vi "Main.vi"(11 "Module Admin":refnum<class "Delacor_lib_QMH_Cloneable Module Admin.lvclass">) -> ()   [LabVIEW 2020, in "Osciloscope.lvlib"]
doc: "This template is based off of the Queued Message Handler design pattern and the Queued Message Handler project template that ships with LabVIEW.\n\nThe main difference is that the queue is private to this module and communication between modules is performed via Broadcast and Request events.\n\nRequest events are wrapped in public API methods and are handled in the Event Handling Loop (EHL) of this VI. Any module can register for Broadcast events sent by this module. The EHL generates messages based on user interface actions.\n\nThe Message Handling Loop (MHL) processes messages generated by the EHL, or by other messages. The messages are string values, so new messages can be added easily to the Message Cases case structure in the MHL. Each message cluster can also provide an optional value for Message Data, which is a variant that can be converted to whatever message-specific data is required.\n_____\nBased on DQMH Project Template 6.0.0.91."
uses:
  Osciloscope.lvlib
  <vilib>/Delacor/Delacor QMH/Libraries/Cloneable Module Admin_class/Delacor_lib_QMH_Cloneable Module Admin.lvclass
  C:/Program Files (x86)/National Instruments/LabVIEW 2020/vi.lib/Delacor/Delacor QMH/Libraries/Module Admin_class/Delacor_lib_QMH_Module Admin.lvclass
  Module Data--cluster.ctl
  Class/Implementaciones/OsciloscopeClass/OsciloscopeClass.lvclass
  <vilib>/Delacor/Delacor QMH/Libraries/Message Queue_class/Delacor_lib_QMH_Message Queue.lvclass/Delacor_lib_QMH_Message Queue.ctl
  <vilib>/Delacor/Delacor QMH/Libraries/Cloneable Module Admin_class/Delacor_lib_QMH_Cloneable Module Admin.lvclass/Delacor_lib_QMH_Cloneable Module Admin.ctl
  Stop Argument--cluster.ctl
  <vilib>/Delacor/Delacor QMH/Libraries/Module Admin_class/Delacor_lib_QMH_Module Admin.lvclass/Delacor_lib_QMH_Module Admin.ctl
  Set Com Port Argument--cluster.ctl
  Inizializate Argument--cluster.ctl
  Init Osciloscope Argument--cluster.ctl
  TypeDefs/InitializeOsciloscope--cluster.ctl
  Close Osciloscope Argument--cluster.ctl
  Auto Setup Osciloscope Argument--cluster.ctl
  Configure Channel Argument--cluster.ctl
  TypeDefs/ConfigurateCahnnel--cluster.ctl
  Reset Osciloscope Argument--cluster.ctl
  Read Waveform Osciloscope Argument--cluster.ctl
  TypeDefs/ReadWaveform--cluster.ctl
  Read Waveform Osciloscope (Reply Payload)--cluster.ctl
  Read Measurement Osciloscope Argument--cluster.ctl
  TypeDefs/ReadMeasurementIn--cluster.ctl
  Read Measurement Osciloscope (Reply Payload)--cluster.ctl
  TypeDefs/ReadMeasurementOut--cluster.ctl
  Read 2 Measurement Channels Osciloscope Argument--cluster.ctl
  TypeDefs/Read2channelsIn--cluster.ctl
  Read 2 Measurement Channels Osciloscope (Reply Payload)--cluster.ctl
  TypeDefs/Read2ChannlesOut.ctl
  <vilib>/Utility/miscctls.llb/LVPointTypeDef.ctl
  Class/Implementaciones/OsciloscopeClass/OsciloscopeClass.lvclass/OsciloscopeClass.ctl
  <vilib>/Delacor/Delacor QMH/Libraries/Message Queue_class/Delacor_lib_QMH_Enqueue Message (Single).vi
  <vilib>/Delacor/Delacor QMH/Libraries/Cloneable Module Admin_class/Delacor_lib_QMH_Get Module ID.vi
  <vilib>/Delacor/Delacor QMH/Libraries/Module Admin_class/Delacor_lib_QMH_Get External Launch.vi
  Class/Implementaciones/OsciloscopeClass/Write Com Port.vi
  <vilib>/Utility/error.llb/Error Cluster From Error Code.vi
  <vilib>/ErrorRing/Error Ring.xnode
  <vilib>/Delacor/Delacor QMH/Libraries/Message Queue_class/Delacor_lib_QMH_Message Queue.lvclass
panel:
  out "error out":errorcluster
  out "Status":string
  in  "Simulate EHL Error":bool
  in  "Simulate MHL Error":bool
  # "Other QMH Modules communicate with this Module via its Public API (wrappers for its Request Events).\n\nThis Module communicates with other Modules via its Broadcast Events.\nAny module that wants to get these messages, just registers for this module's Broadcast events."
  # "This template is for the Delacor Modified Queued Message Handler design pattern.\n\nSee the block diagram for more information on how to use this template."
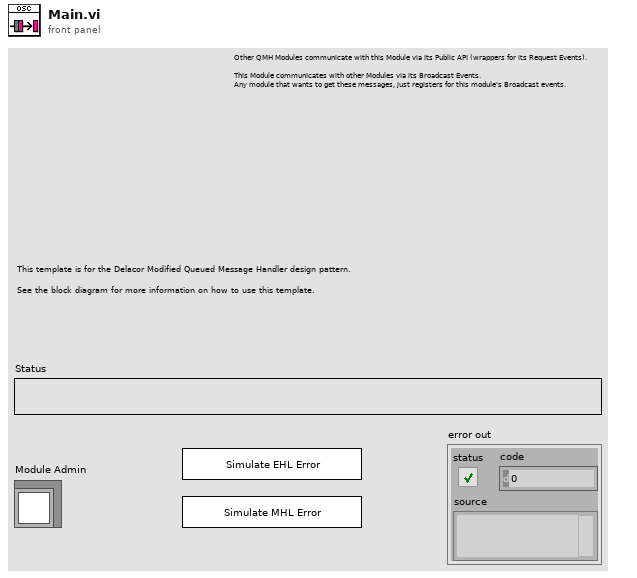
[diagram p1: front panel]
types:
  T1 = typedef "Osciloscope.lvlib/Request Events--cluster.ctl" = cluster{"Stop Module":refnum<user-event>, "Show Panel":refnum<user-event>, "Hide Panel":refnum<user-event>, "Show Diagram":refnum<user-event>, "Get Module Execution Status":refnum<user-event>, "Set Com Port":refnum<user-event>, "Inizializate":refnum<user-event>, "Init Osciloscope":refnum<user-event>, "Close Osciloscope":refnum<user-event>, "Auto Setup Osciloscope":refnum<user-event>, "Configure Channel":refnum<user-event>, "Reset Osciloscope":refnum<user-event>, "Read Waveform Osciloscope":refnum<user-event>, "Read Measurement Osciloscope":refnum<user-event>, "Read 2 Measurement Channels Osciloscope":refnum<user-event>}
  T2 = typedef "Osciloscope.lvlib/Module Data--cluster.ctl" = cluster{"Status":string, "OsciloscopeClass.lvclass":refnum<class "OsciloscopeClass.lvclass">}
  T3 = enum32{"invalid lock state", "Not Locked", "Locked (No Password)", "Password-protected"}
  T4 = typedef "Osciloscope.lvlib/Stop Argument--cluster.ctl" = cluster{"Module ID":i32, "Origin":string, "Exit via Stop Module Req?":bool, "Wait for Module to stop?":bool}
  T5 = typedef "Osciloscope.lvlib/Set Com Port Argument--cluster.ctl" = cluster{"Module ID":i32, "Com Port":refnum<visa-resource-name>}
  T6 = typedef "Osciloscope.lvlib/Inizializate Argument--cluster.ctl" = cluster{"Module ID":i32, "Osciloscope":string}
  T7 = typedef "Osciloscope.lvlib/Init Osciloscope Argument--cluster.ctl" = cluster{"Module ID":i32, "Boolean":bool, "Initialize--cluster":T8}
  T8 = typedef "InitializeOsciloscope--cluster.ctl" = cluster{"TEKTRONIX-INITIALIZE":cluster{"ID Query? (T: Yes)":bool, "Reset? (T: Yes)":bool, "Serial-Configuration":cluster{"Baud Rate":u32, "Parity":u16, "Stop Bits":u16, "Flow Control":u16}}, "EDU-X-1200A- INITIALIZE":cluster{"Reset (True)":bool, "ID Query (True)":bool}}
  T9 = typedef "Osciloscope.lvlib/Close Osciloscope Argument--cluster.ctl" = cluster{"Module ID":i32, "Boolean":bool}
  T10 = typedef "Osciloscope.lvlib/Auto Setup Osciloscope Argument--cluster.ctl" = cluster{"Module ID":i32, "Boolean":bool}
  T11 = typedef "Osciloscope.lvlib/Configure Channel Argument--cluster.ctl" = cluster{"Module ID":i32, "Configurate Channel--cluster":T12}
  T12 = typedef "ConfigurateCahnnel--cluster.ctl" = cluster{"Tektronix":cluster{"Enable Channel (True)":bool, "Channel (0: Channel 1)":i32, "Vertical Coupling (1: DC)":i32, "Probe Attenuation (10: 10X)":i32, "Vertical Range (10.0 V/div)":dbl, "Vertical Offset (0.0 divs)":dbl, "Bandwidth (0: MAX Bandwidth)":i32}, "EDU-X-1002A":cluster{"Vertical Scale (5.0 V)":dbl, "Impedance (0: 1 MOhm)":i32, "Channel Name (0: Channel 1)":i32, "Coupling (1: DC)":i32, "Vertical Range (40.0 V)":dbl, "Vertical Offset (0.0)":dbl, "Probe Attenuation (1.0)":dbl, "Vertical Setting (1: Vertical Range)":i32}}
  T13 = typedef "Osciloscope.lvlib/Reset Osciloscope Argument--cluster.ctl" = cluster{"Module ID":i32, "Boolean":bool}
  T14 = typedef "Osciloscope.lvlib/Read Waveform Osciloscope Argument--cluster.ctl" = cluster{"Module ID":i32, "ReadWaveform":T15, "Wait Notifier":refnum<notifier>, "wait for reply":bool}
  T15 = typedef "ReadWaveform--cluster.ctl" = cluster{"TEKTRONIX READ-WAVEFORM 2":cluster{"Source (0: Channel 1)":u16, "Timeout (10000 ms) 2":u32}, "EDU-X-1200A- READ-WAVEFORM":cluster{"Bind Source Channel (2: None)":i32, "Timeout (10000 ms)":u32, "Source Channel (0: Channel 1)":i32}}
  T16 = typedef "Osciloscope.lvlib/Read Measurement Osciloscope Argument--cluster.ctl" = cluster{"Module ID":i32, "Read Measurement In":T17, "Wait Notifier":refnum<notifier>, "wait for reply":bool}
  T17 = typedef "ReadMeasurementIn--cluster.ctl" = cluster{"TEKTRONIX- READ-IN":cluster{"Channel (1: Channel 1)":i32, "Measurement Type (0: Frequency)":i32}, "EDU-X-1200A- READ-IN":cluster{"Slope Type (0: Positive)":i32, "Measurement Type (0: Peak-Peak)":i32, "Occurrence Value (1)":i32, "Vertical Cross Value (0)":dbl}}
  T18 = typedef "Osciloscope.lvlib/Read 2 Measurement Channels Osciloscope Argument--cluster.ctl" = cluster{"Module ID":i32, "Read 2 channels In":T19, "Wait Notifier":refnum<notifier>, "wait for reply":bool}
  T19 = typedef "Read2channelsIn--cluster.ctl" = cluster{"TEKTRONIX- READ-CHANNELS-IN":cluster{"Channel 1 (1: Channel 1)":i32, "Channel 2 (2: Channel 2)":i32, "Measurement Type (0: Phase)":i32}, "EDU-X-1200A- READ-CHANNELS-IN":cluster{"Timeout (10000 ms)":u32, "Channels":i32[]}}
  T20 = typedef "LVPointTypeDef.ctl" = cluster{"Horizontal":i16, "Vertical":i16}
  T21 = enum32{"Invalid", "Standard", "Closed", "Hidden", "Minimized", "Maximized"}
  T22 = typedef "Osciloscope.lvlib/Read Waveform Osciloscope (Reply Payload)--cluster.ctl" = cluster{"Waveform Graph":dbl[], "Read Waveform Osciloscope_error":errorcluster}
  T23 = typedef "Osciloscope.lvlib/Read Measurement Osciloscope (Reply Payload)--cluster.ctl" = cluster{"Read measurement Out":T24, "Read Measurement Osciloscope_error":errorcluster}
  T24 = typedef "ReadMeasurementOut--cluster.ctl" = cluster{"Tektronix-1200A-READ-OUT":cluster{"Units":string, "Measurement":dbl}, "EDU-X-1200A- READ-OUT":cluster{"Measurement":dbl}}
  T25 = typedef "Osciloscope.lvlib/Read 2 Measurement Channels Osciloscope (Reply Payload)--cluster.ctl" = cluster{"Read 2 channels Out":T26, "Read 2 Measurement Channels Osciloscope_error":errorcluster}
  T26 = typedef "Read2ChannlesOut.ctl" = cluster{"TEKTRONIX READ-CHANNELS-OUT ":cluster{"Units":string, "Measurement":dbl}, "EDU-X-1200A- READ-CHANNELS-OUT":cluster{"Measurements":dbl[]}}
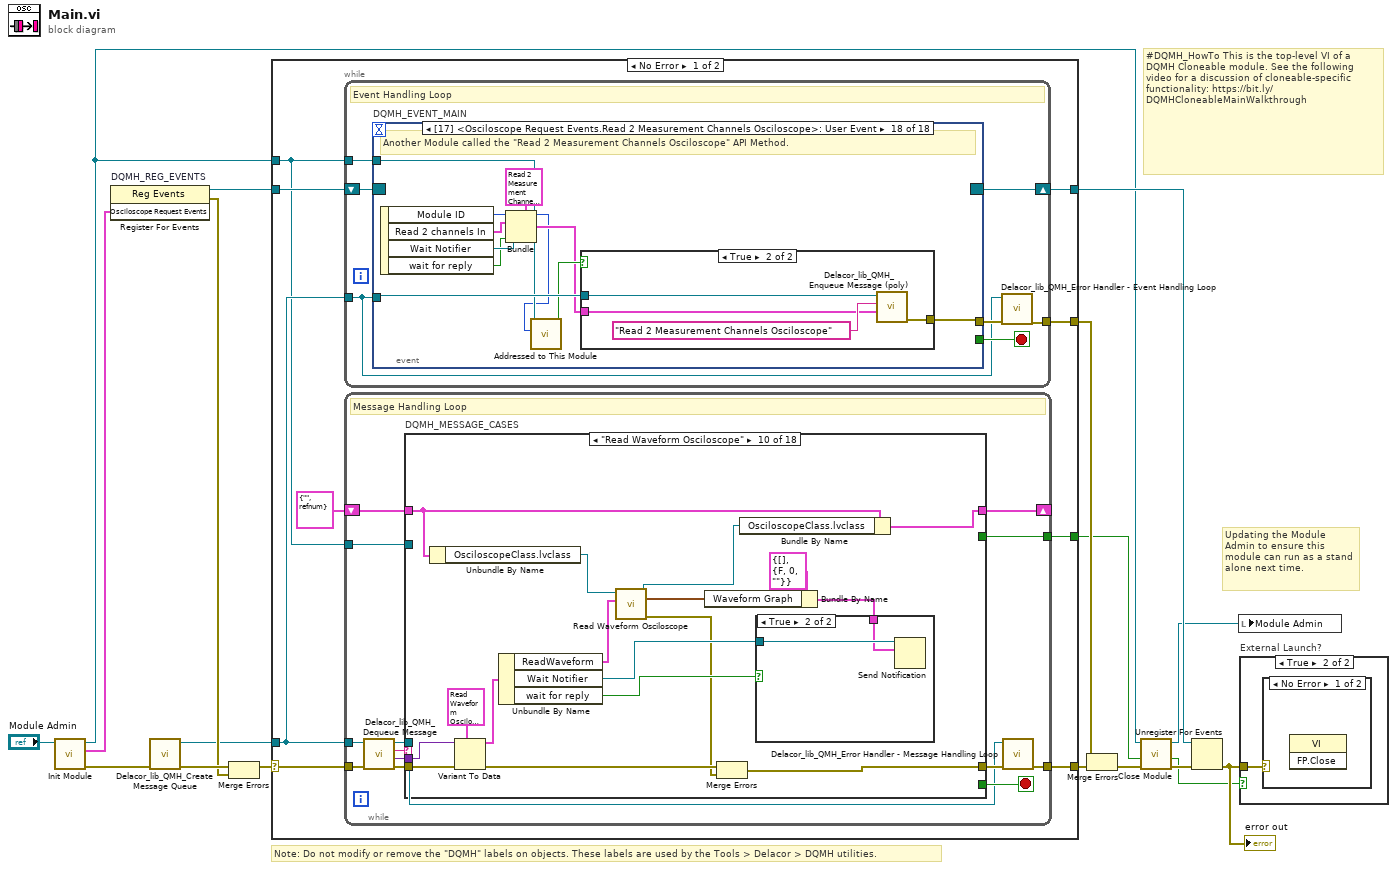
[diagram p0: block diagram]
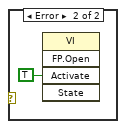
[diagram p3: hidden frame]
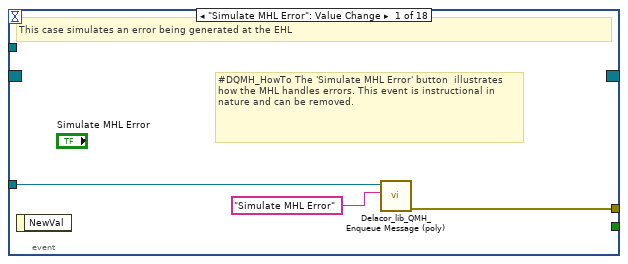
[diagram p4: hidden frame]
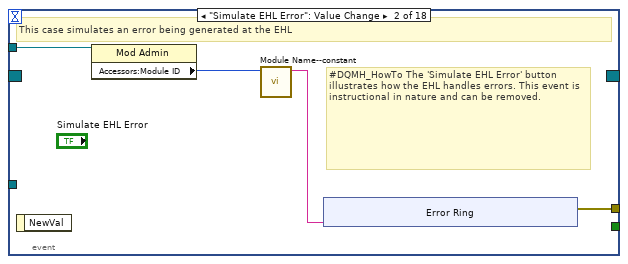
[diagram p5: hidden frame]
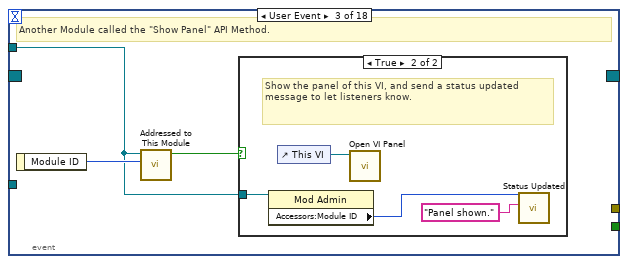
[diagram p6: hidden frame]
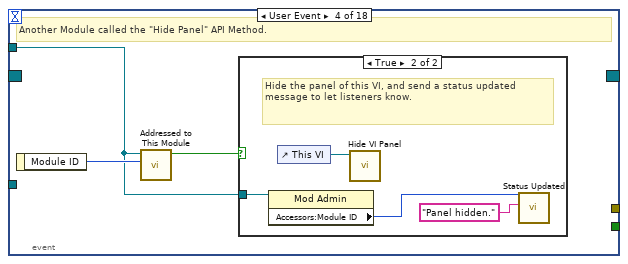
[diagram p8: hidden frame]
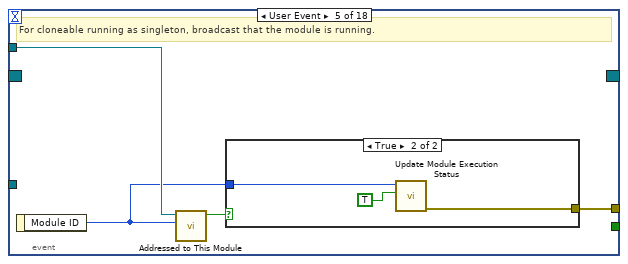
[diagram p10: hidden frame]
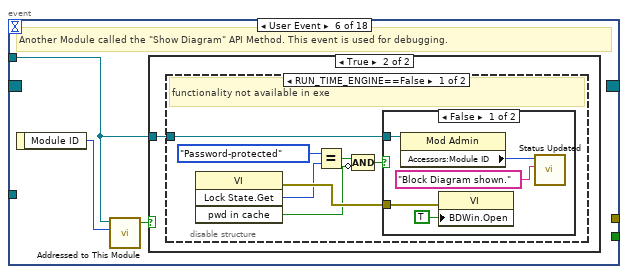
[diagram p12: hidden frame]
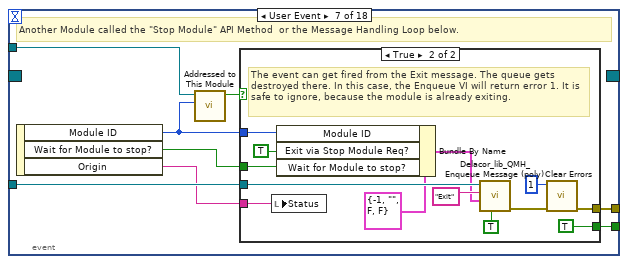
[diagram p16: hidden frame]
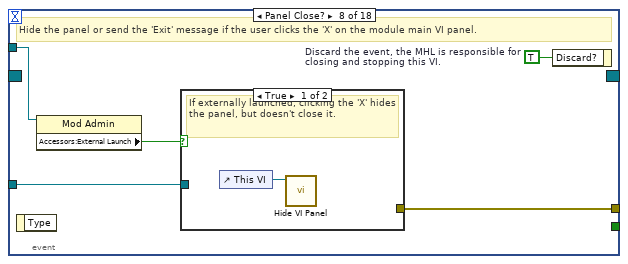
[diagram p18: hidden frame]
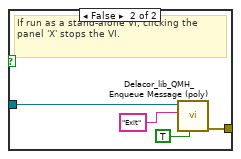
[diagram p19: hidden frame]
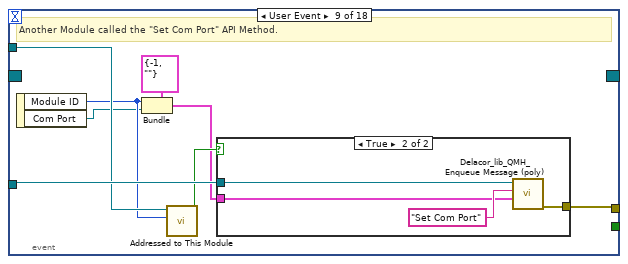
[diagram p20: hidden frame]
diagram:
  # "#DQMH_HowTo This is the top-level VI of a DQMH Cloneable module. See the following video for a discussion of cloneable-specific functionality: https://bit.ly/DQMHCloneableMainWalkthrough"
  # "Note: Do not modify or remove the \"DQMH\" labels on objects. These labels are used by the Tools > Delacor > DQMH utilities."
  # "Updating the Module Admin to ensure this module can run as a stand alone next time."
  n1 = call "Init Module.vi"("Cloneable Module Admin in"="Module Admin") -> ("error out"=w15:errorcluster, "Osciloscope Request Events"=w7:T1, "Cloneable Module Admin out"=w4:refnum<class "Delacor_lib_QMH_Cloneable Module Admin.lvclass">)  [unwired: 8 in]
  n2 = register-events "DQMH_REG_EVENTS"(w7) -> (reference out=w8:refnum<event-registration>, error out=w10:errorcluster)  [unwired: 2 in]
  n3 = call <vilib>:"Delacor_lib_QMH_Create Message Queue.vi"("error in"=w15) -> ("error out"=w12:errorcluster, "Message Queue"=w6:refnum<class "Delacor_lib_QMH_Message Queue.lvclass">)  [unwired: 9 in]
  n4 = Merge Errors(w12, w10) -> (w11:errorcluster)
  n5 = case shown="No Error" w11 {
    selector: w11 -> [w25 w475]
    tunnel: [w27 w474] -> w16
    tunnel: [w24 w482] -> w9
    tunnel: w8 -> [w22 w482]
    tunnel: w6 -> [w21 w473]
    tunnel: [w26 _] -> w17
    tunnel: w4 -> [w20 w478]
    tunnel: [w19 _] -> w2
    frame No Error {
      n6 = while {
        tunnel: w21 -> [w28]
        shift-right: [w31] -> w24
        shift-left: w22 -> [w32]
        tunnel: [w33] -> w26
        tunnel: w20 -> [w29]
        stop <- w30 stop-if-true
        # "Event Handling Loop"
        n7 = event "DQMH_EVENT_MAIN" shown="[17] <Osciloscope Request Events.Read 2 Measurement Channels Osciloscope>: User Event" {
          selector: w32 -> [_ _ _ _ _ _ _ _ _ _ _ _ _ _ _ _ _ _]
          dyn-events: [_ _ _ _ _ _ _ _ _ _ _ _ _ _ _ _ _ _] -> w31
          timeout: _ -> [_ _ _ _ _ _ _ _ _ _ _ _ _ _ _ _ _ _]
          tunnel: [_ _ _ _ _ _ w89 _ _ _ _ _ _ _ _ _ _ _] -> w30
          tunnel: w28 -> [w36 _ _ _ _ _ w92 w108 w124 w136 w149 w161 w173 w185 w197 w211 w225 w239]
          tunnel: [w37 w41 _ _ w66 _ w93 w111 w117 w129 w142 w154 w166 w178 w190 w202 w216 w230] -> w34
          tunnel: w29 -> [_ w40 w49 w56 w64 w70 w91 w109 w122 w134 w147 w159 w171 w183 w195 w209 w223 w237]
          event "Simulate MHL Error": Value Change {
            # "#DQMH_HowTo The 'Simulate MHL Error' button  illustrates how the MHL handles errors. This event is instructional in nature and can be removed."
            # "This case simulates an error being generated at the EHL"
            n8 = event-data() -> ()  [unwired: 1 in, 1 out]
            n9 = call-poly <vilib>:"Delacor_lib_QMH_Enqueue Message (poly).vi"("Message"="Simulate MHL Error", "Message Queue in"=w36) -> ("error out"=w37:errorcluster)  [unwired: 8 in, 1 out]
          }
          event "Simulate EHL Error": Value Change {
            # "#DQMH_HowTo The 'Simulate EHL Error' button  illustrates how the EHL handles errors. This event is instructional in nature and can be removed."
            # "This case simulates an error being generated at the EHL"
            n10 = event-data() -> ()  [unwired: 1 in, 1 out]
            n11 = property class="Mod Admin"(reference=w40) -> ("Accessors:Module ID"=w39:i32)  [unwired: 1 in, 2 out]
            n12 = call "Module Name--constant.vi"("Module ID"=w39) -> ("Module Name"=w38:string)  [unwired: 10 in]
            n13 = xnode "Error Ring"("parameter 0"=w38) -> ("error out"=w41:errorcluster)
          }
          event User Event {
            # "Another Module called the \"Show Panel\" API Method."
            n14 = event-data() -> ("Module ID"=w50:i32)  [unwired: 1 in]
            n15 = call "Addressed to This Module.vi"("Module ID from Argument"=w50, "Module Admin"=w49) -> ("Addressed to this instance?"=w51:bool)  [unwired: 8 in, 1 out]
            n16 = case shown="True" w51 {
              tunnel: w49 -> [_ w53]
              frame False {
              }
              frame True {
                # "Show the panel of this VI, and send a status updated message to let listeners know."
                n17 = property class="Mod Admin"(reference=w53) -> ("Accessors:Module ID"=w52:i32)  [unwired: 1 in, 2 out]
                n18 = control-ref of="This VI"() -> (w55:refnum<vi>)
                n19 = call "Open VI Panel.vi"("VI"=w55) -> ()  [unwired: 10 in, 1 out]
                n20 = call "Status Updated.vi"("Status"="Panel shown." ("format string"), "Module ID"=w52) -> ()  [unwired: 9 in, 1 out]
              }
            }
          }
          event User Event {
            # "Another Module called the \"Hide Panel\" API Method."
            n21 = event-data() -> ("Module ID"=w57:i32)  [unwired: 1 in]
            n22 = call "Addressed to This Module.vi"("Module ID from Argument"=w57, "Module Admin"=w56) -> ("Addressed to this instance?"=w58:bool)  [unwired: 8 in, 1 out]
            n23 = case shown="True" w58 {
              tunnel: w56 -> [_ w60]
              frame False {
              }
              frame True {
                # "Hide the panel of this VI, and send a status updated message to let listeners know."
                n24 = property class="Mod Admin"(reference=w60) -> ("Accessors:Module ID"=w59:i32)  [unwired: 1 in, 2 out]
                n25 = control-ref of="This VI"() -> (w62:refnum<vi>)
                n26 = call "Hide VI Panel.vi"("VI"=w62) -> ()  [unwired: 10 in, 1 out]
                n27 = call "Status Updated.vi"("Status"="Panel hidden." ("format string"), "Module ID"=w59) -> ()  [unwired: 9 in, 1 out]
              }
            }
          }
          event User Event {
            # "For cloneable running as singleton, broadcast that the module is running."
            n28 = event-data() -> ("Module ID"=w63:i32)  [unwired: 1 in]
            n29 = call "Addressed to This Module.vi"("Module ID from Argument"=w63, "Module Admin"=w64) -> ("Addressed to this instance?"=w65:bool)  [unwired: 8 in, 1 out]
            n30 = case shown="True" w65 {
              tunnel: [_ w69] -> w66
              tunnel: w63 -> [_ w68]
              frame False {
              }
              frame True {
                n31 = call "Update Module Execution Status.vi"("Running?"=TRUE, "Module ID"=w68) -> ("error out"=w69:errorcluster)  [unwired: 9 in]
              }
            }
          }
          event User Event {
            # "Another Module called the \"Show Diagram\" API Method. This event is used for debugging."
            n32 = event-data() -> ("Module ID"=w71:i32)  [unwired: 1 in]
            n33 = call "Addressed to This Module.vi"("Module ID from Argument"=w71, "Module Admin"=w70) -> ("Addressed to this instance?"=w72:bool)  [unwired: 8 in, 1 out]
            n34 = case shown="True" w72 {
              tunnel: w70 -> [_ w73]
              frame False {
              }
              frame True {
                n35 = disable-structure shown="RUN_TIME_ENGINE==False" {
                  disable-tunnel: w73 -> [w74 _]
                  frame condition #0 (active) {
                    # "functionality not available in exe"
                    n36 = invoke class="VI" method="Lock State.Get"() -> (error out=w80:errorcluster, "Get Lock State"=w79:T3, "pwd in cache"=w76:bool)  [unwired: 4 in, 1 out]
                    n37 = Equal?(x=T3."Password-protected", y=w79) -> (x = y?=w77:bool)
                    n38 = Compound Arithmetic op=AND(w77, invert w76) -> (w75:bool)
                    n39 = case shown="False" w75 {
                      tunnel: w80 -> [w85 _]
                      tunnel: w74 -> [w82 _]
                      frame False {
                        n40 = property class="Mod Admin"(reference=w82) -> ("Accessors:Module ID"=w81:i32)  [unwired: 1 in, 2 out]
                        n41 = property class="VI"(error in=w85, "BDWin.Open"=TRUE ("Block Diagram Window:Open")) -> ()  [unwired: 1 in, 2 out]
                        n42 = call "Status Updated.vi"("Status"="Block Diagram shown." ("format string"), "Module ID"=w81) -> ()  [unwired: 9 in, 1 out]
                      }
                      frame True {
                        # "Password-protected VI, and the password is not in the cache. Do not show the diagram."
                      }
                    }
                  }
                  frame condition #1 {
                  }
                }
              }
            }
          }
          event User Event {
            # "Another Module called the \"Stop Module\" API Method  or the Message Handling Loop below."
            n43 = event-data() -> ("Module ID"=w87:i32, "Wait for Module to stop?"=w88:bool, "Origin"=w86:string)  [unwired: 1 in]
            n44 = call "Addressed to This Module.vi"("Module ID from Argument"=w87, "Module Admin"=w91) -> ("Addressed to this instance?"=w90:bool)  [unwired: 8 in, 1 out]
            n45 = case shown="True" w90 {
              tunnel: [_ w105] -> w93
              tunnel: w92 -> [_ w101]
              tunnel: [_ TRUE] -> w89
              tunnel: w88 -> [_ w96]
              tunnel: w87 -> [_ w98]
              tunnel: w86 -> [_ w94]
              frame False {
              }
              frame True {
                # "The event can get fired from the Exit message. The queue gets destroyed there. In this case, the Enqueue VI will return error 1. It is safe to ignore, because the module is already exiting."
                n46 = local write "Status"(w94) -> ()
                n47 = Bundle By Name(cluster=T4 {"Module ID"=-1, "Origin"="", "Exit via Stop Module Req?"=FALSE, "Wait for Module to stop?"=FALSE} ("Stop Argument"), "Module ID"=w98, "Exit via Stop Module Req?"=TRUE, "Wait for Module to stop?"=w96) -> (w95:T4)
                n48 = call-poly <vilib>:"Delacor_lib_QMH_Enqueue Message (poly).vi"("Priority Message? (F)"=TRUE, "Message Data"=w95, "Message"="Exit", "Message Queue in"=w101) -> ("error out"=w106:errorcluster)  [unwired: 6 in, 1 out]
                n49 = call <vilib>:"Clear Errors.vi"("error in (no error)"=w106, "specific error code to clear (0: all)"=1) -> ("error out"=w105:errorcluster)  [unwired: 4 in, 1 out]
              }
            }
          }
          event Panel Close? {
            w110 = TRUE  # Discard the event, the MHL is responsible for closing and stopping this VI.
            # "Hide the panel or send the 'Exit' message if the user clicks the 'X' on the module main VI panel."
            n50 = event-data() -> ()  [unwired: 1 in, 1 out]
            n51 = property class="Mod Admin"(reference=w109) -> ("Accessors:External Launch"=w107:bool)  [unwired: 1 in, 2 out]
            n52 = case shown="True" w107 {
              tunnel: w108 -> [_ w115]
              tunnel: [_ w116] -> w111
              frame True {
                # "If externally launched, clicking the 'X' hides the panel, but doesn't close it."
                n53 = control-ref of="This VI"() -> (w112:refnum<vi>)
                n54 = call "Hide VI Panel.vi"("VI"=w112) -> ()  [unwired: 10 in, 1 out]
              }
              frame False {
                # "If run as a stand-alone VI, clicking the panel 'X' stops the VI."
                n55 = call-poly <vilib>:"Delacor_lib_QMH_Enqueue Message (poly).vi"("Priority Message? (F)"=TRUE, "Message"="Exit", "Message Queue in"=w115) -> ("error out"=w116:errorcluster)  [unwired: 7 in, 1 out]
              }
            }
            n56 = event-data("Discard?"=w110) -> ()  [unwired: 1 in, 1 out]
          }
          event User Event {
            # "Another Module called the \"Set Com Port\" API Method."
            n57 = event-data() -> ("Module ID"=w119:i32, "Com Port"=w118:refnum<visa-resource-name>)  [unwired: 1 in]
            n58 = Bundle(cluster=T5 {"Module ID"=-1, "Com Port"=""} ("Set Com Port Argument"), "Module ID"=w119, "Com Port"=w118) -> (w120:T5)
            n59 = call "Addressed to This Module.vi"("Module ID from Argument"=w119, "Module Admin"=w122) -> ("Addressed to this instance?"=w123:bool)  [unwired: 8 in, 1 out]
            n60 = case shown="True" w123 {
              tunnel: w124 -> [_ w128]
              tunnel: w120 -> [_ w126]
              tunnel: [_ w125] -> w117
              frame False {
              }
              frame True {
                n61 = call-poly <vilib>:"Delacor_lib_QMH_Enqueue Message (poly).vi"("Message Data"=w126, "Message"="Set Com Port", "Message Queue in"=w128) -> ("error out"=w125:errorcluster)  [unwired: 7 in, 1 out]
              }
            }
          }
          event User Event {
            # "Another Module called the \"Inizializate\" API Method."
            n62 = event-data() -> ("Module ID"=w131:i32, "Osciloscope"=w130:string)  [unwired: 1 in]
            n63 = Bundle(cluster=T6 {"Module ID"=-1, "Osciloscope"=""} ("Inizializate Argument"), "Module ID"=w131, "Osciloscope"=w130) -> (w132:T6)
            n64 = call "Addressed to This Module.vi"("Module ID from Argument"=w131, "Module Admin"=w134) -> ("Addressed to this instance?"=w135:bool)  [unwired: 8 in, 1 out]
            n65 = case shown="True" w135 {
              tunnel: w136 -> [_ w140]
              tunnel: w132 -> [_ w138]
              tunnel: [_ w137] -> w129
              frame False {
              }
              frame True {
                n66 = call-poly <vilib>:"Delacor_lib_QMH_Enqueue Message (poly).vi"("Message Data"=w138, "Message"="Inizializate", "Message Queue in"=w140) -> ("error out"=w137:errorcluster)  [unwired: 7 in, 1 out]
              }
            }
          }
          event User Event {
            # "Another Module called the \"Init Osciloscope\" API Method."
            n67 = event-data() -> ("Module ID"=w144:i32, "Boolean"=w143:bool, "Initialize--cluster"=w141:T8)  [unwired: 1 in]
            n68 = Bundle(cluster=T7 {"Module ID"=-1, "Boolean"=FALSE, "Initialize--cluster"={"TEKTRONIX-INITIALIZE"={"ID Query? (T: Yes)"=TRUE, "Reset? (T: Yes)"=TRUE, "Serial-Configuration"={"Baud Rate"=9600, "Parity"=0, "Stop Bits"=10, "Flow Control"=2}}, "EDU-X-1200A- INITIALIZE"={"Reset (True)"=TRUE, "ID Query (True)"=TRUE}}} ("Init Osciloscope Argument"), "Module ID"=w144, "Boolean"=w143, "Initialize--cluster"=w141) -> (w145:T7)
            n69 = call "Addressed to This Module.vi"("Module ID from Argument"=w144, "Module Admin"=w147) -> ("Addressed to this instance?"=w148:bool)  [unwired: 8 in, 1 out]
            n70 = case shown="True" w148 {
              tunnel: w149 -> [_ w153]
              tunnel: w145 -> [_ w151]
              tunnel: [_ w150] -> w142
              frame False {
              }
              frame True {
                n71 = call-poly <vilib>:"Delacor_lib_QMH_Enqueue Message (poly).vi"("Message Data"=w151, "Message"="Init Osciloscope", "Message Queue in"=w153) -> ("error out"=w150:errorcluster)  [unwired: 7 in, 1 out]
              }
            }
          }
          event User Event {
            # "Another Module called the \"Close Osciloscope\" API Method."
            n72 = event-data() -> ("Module ID"=w156:i32, "Boolean"=w155:bool)  [unwired: 1 in]
            n73 = Bundle(cluster=T9 {"Module ID"=-1, "Boolean"=FALSE} ("Close Osciloscope Argument"), "Module ID"=w156, "Boolean"=w155) -> (w157:T9)
            n74 = call "Addressed to This Module.vi"("Module ID from Argument"=w156, "Module Admin"=w159) -> ("Addressed to this instance?"=w160:bool)  [unwired: 8 in, 1 out]
            n75 = case shown="True" w160 {
              tunnel: w161 -> [_ w165]
              tunnel: w157 -> [_ w163]
              tunnel: [_ w162] -> w154
              frame False {
              }
              frame True {
                n76 = call-poly <vilib>:"Delacor_lib_QMH_Enqueue Message (poly).vi"("Message Data"=w163, "Message"="Close Osciloscope", "Message Queue in"=w165) -> ("error out"=w162:errorcluster)  [unwired: 7 in, 1 out]
              }
            }
          }
          event User Event {
            # "Another Module called the \"Auto Setup Osciloscope\" API Method."
            n77 = event-data() -> ("Module ID"=w168:i32, "Boolean"=w167:bool)  [unwired: 1 in]
            n78 = Bundle(cluster=T10 {"Module ID"=-1, "Boolean"=FALSE} ("Auto Setup Osciloscope Argument"), "Module ID"=w168, "Boolean"=w167) -> (w169:T10)
            n79 = call "Addressed to This Module.vi"("Module ID from Argument"=w168, "Module Admin"=w171) -> ("Addressed to this instance?"=w172:bool)  [unwired: 8 in, 1 out]
            n80 = case shown="True" w172 {
              tunnel: w173 -> [_ w177]
              tunnel: w169 -> [_ w175]
              tunnel: [_ w174] -> w166
              frame False {
              }
              frame True {
                n81 = call-poly <vilib>:"Delacor_lib_QMH_Enqueue Message (poly).vi"("Message Data"=w175, "Message"="Auto Setup Osciloscope", "Message Queue in"=w177) -> ("error out"=w174:errorcluster)  [unwired: 7 in, 1 out]
              }
            }
          }
          event User Event {
            # "Another Module called the \"Configure Channel\" API Method."
            n82 = event-data() -> ("Module ID"=w180:i32, "Configurate Channel--cluster"=w179:T12)  [unwired: 1 in]
            n83 = Bundle(cluster=T11 {"Module ID"=-1, "Configurate Channel--cluster"={"Tektronix"={"Enable Channel (True)"=TRUE, "Channel (0: Channel 1)"=0, "Vertical Coupling (1: DC)"=1, "Probe Attenuation (10: 10X)"=10, "Vertical Range (10.0 V/div)"=10.0, "Vertical Offset (0.0 divs)"=0.0, "Bandwidth (0: MAX Bandwidth)"=0}, "EDU-X-1002A"={"Vertical Scale (5.0 V)"=5.0, "Impedance (0: 1 MOhm)"=0, "Channel Name (0: Channel 1)"=0, "Coupling (1: DC)"=1, "Vertical Range (40.0 V)"=40.0, "Vertical Offset (0.0)"=0.0, "Probe Attenuation (1.0)"=1.0, "Vertical Setting (1: Vertical Range)"=1}}} ("Configure Channel Argument"), "Module ID"=w180, "Configurate Channel--cluster"=w179) -> (w181:T11)
            n84 = call "Addressed to This Module.vi"("Module ID from Argument"=w180, "Module Admin"=w183) -> ("Addressed to this instance?"=w184:bool)  [unwired: 8 in, 1 out]
            n85 = case shown="True" w184 {
              tunnel: w185 -> [_ w189]
              tunnel: w181 -> [_ w187]
              tunnel: [_ w186] -> w178
              frame False {
              }
              frame True {
                n86 = call-poly <vilib>:"Delacor_lib_QMH_Enqueue Message (poly).vi"("Message Data"=w187, "Message"="Configure Channel", "Message Queue in"=w189) -> ("error out"=w186:errorcluster)  [unwired: 7 in, 1 out]
              }
            }
          }
          event User Event {
            # "Another Module called the \"Reset Osciloscope\" API Method."
            n87 = event-data() -> ("Module ID"=w192:i32, "Boolean"=w191:bool)  [unwired: 1 in]
            n88 = Bundle(cluster=T13 {"Module ID"=-1, "Boolean"=FALSE} ("Reset Osciloscope Argument"), "Module ID"=w192, "Boolean"=w191) -> (w193:T13)
            n89 = call "Addressed to This Module.vi"("Module ID from Argument"=w192, "Module Admin"=w195) -> ("Addressed to this instance?"=w196:bool)  [unwired: 8 in, 1 out]
            n90 = case shown="True" w196 {
              tunnel: w197 -> [_ w201]
              tunnel: w193 -> [_ w199]
              tunnel: [_ w198] -> w190
              frame False {
              }
              frame True {
                n91 = call-poly <vilib>:"Delacor_lib_QMH_Enqueue Message (poly).vi"("Message Data"=w199, "Message"="Reset Osciloscope", "Message Queue in"=w201) -> ("error out"=w198:errorcluster)  [unwired: 7 in, 1 out]
              }
            }
          }
          event User Event {
            # "Another Module called the \"Read Waveform Osciloscope\" API Method."
            n92 = event-data() -> ("Module ID"=w206:i32, "ReadWaveform"=w205:T15, "Wait Notifier"=w204:refnum<notifier>, "wait for reply"=w203:bool)  [unwired: 1 in]
            n93 = Bundle(cluster=T14 {"Module ID"=-1, "ReadWaveform"={"TEKTRONIX READ-WAVEFORM 2"={"Source (0: Channel 1)"=0, "Timeout (10000 ms) 2"=10000}, "EDU-X-1200A- READ-WAVEFORM"={"Bind Source Channel (2: None)"=2, "Timeout (10000 ms)"=10000, "Source Channel (0: Channel 1)"=0}}, "Wait Notifier"=refnum, "wait for reply"=FALSE} ("Read Waveform Osciloscope Argument"), "Module ID"=w206, "ReadWaveform"=w205, "Wait Notifier"=w204, "wait for reply"=w203) -> (w207:T14)
            n94 = call "Addressed to This Module.vi"("Module ID from Argument"=w206, "Module Admin"=w209) -> ("Addressed to this instance?"=w210:bool)  [unwired: 8 in, 1 out]
            n95 = case shown="True" w210 {
              tunnel: w211 -> [_ w215]
              tunnel: w207 -> [_ w213]
              tunnel: [_ w212] -> w202
              frame False {
              }
              frame True {
                n96 = call-poly <vilib>:"Delacor_lib_QMH_Enqueue Message (poly).vi"("Message Data"=w213, "Message"="Read Waveform Osciloscope", "Message Queue in"=w215) -> ("error out"=w212:errorcluster)  [unwired: 7 in, 1 out]
              }
            }
          }
          event User Event {
            # "Another Module called the \"Read Measurement Osciloscope\" API Method."
            n97 = event-data() -> ("Module ID"=w220:i32, "Read Measurement In"=w219:T17, "Wait Notifier"=w218:refnum<notifier>, "wait for reply"=w217:bool)  [unwired: 1 in]
            n98 = Bundle(cluster=T16 {"Module ID"=-1, "Read Measurement In"={"TEKTRONIX- READ-IN"={"Channel (1: Channel 1)"=1, "Measurement Type (0: Frequency)"=0}, "EDU-X-1200A- READ-IN"={"Slope Type (0: Positive)"=0, "Measurement Type (0: Peak-Peak)"=0, "Occurrence Value (1)"=1, "Vertical Cross Value (0)"=0.0}}, "Wait Notifier"=refnum, "wait for reply"=FALSE} ("Read Measurement Osciloscope Argument"), "Module ID"=w220, "Read Measurement In"=w219, "Wait Notifier"=w218, "wait for reply"=w217) -> (w221:T16)
            n99 = call "Addressed to This Module.vi"("Module ID from Argument"=w220, "Module Admin"=w223) -> ("Addressed to this instance?"=w224:bool)  [unwired: 8 in, 1 out]
            n100 = case shown="True" w224 {
              tunnel: w225 -> [_ w229]
              tunnel: w221 -> [_ w227]
              tunnel: [_ w226] -> w216
              frame False {
              }
              frame True {
                n101 = call-poly <vilib>:"Delacor_lib_QMH_Enqueue Message (poly).vi"("Message Data"=w227, "Message"="Read Measurement Osciloscope", "Message Queue in"=w229) -> ("error out"=w226:errorcluster)  [unwired: 7 in, 1 out]
              }
            }
          }
          event User Event {
            # "Another Module called the \"Read 2 Measurement Channels Osciloscope\" API Method."
            n102 = event-data() -> ("Module ID"=w234:i32, "Read 2 channels In"=w233:T19, "Wait Notifier"=w232:refnum<notifier>, "wait for reply"=w231:bool)  [unwired: 1 in]
            n103 = Bundle(cluster=T18 {"Module ID"=-1, "Read 2 channels In"={"TEKTRONIX- READ-CHANNELS-IN"={"Channel 1 (1: Channel 1)"=1, "Channel 2 (2: Channel 2)"=2, "Measurement Type (0: Phase)"=0}, "EDU-X-1200A- READ-CHANNELS-IN"={"Timeout (10000 ms)"=10000, "Channels"=[]}}, "Wait Notifier"=refnum, "wait for reply"=FALSE} ("Read 2 Measurement Channels Osciloscope Argument"), "Module ID"=w234, "Read 2 channels In"=w233, "Wait Notifier"=w232, "wait for reply"=w231) -> (w235:T18)
            n104 = call "Addressed to This Module.vi"("Module ID from Argument"=w234, "Module Admin"=w237) -> ("Addressed to this instance?"=w238:bool)  [unwired: 8 in, 1 out]
            n105 = case shown="True" w238 {
              tunnel: w239 -> [_ w243]
              tunnel: w235 -> [_ w241]
              tunnel: [_ w240] -> w230
              frame False {
              }
              frame True {
                n106 = call-poly <vilib>:"Delacor_lib_QMH_Enqueue Message (poly).vi"("Message Data"=w241, "Message"="Read 2 Measurement Channels Osciloscope", "Message Queue in"=w243) -> ("error out"=w240:errorcluster)  [unwired: 7 in, 1 out]
              }
            }
          }
        }
        n107 = call-dynamic "Delacor_lib_QMH_Error Handler - Event Handling Loop.vi"("error in"=w34, "Message Queue in"=w28) -> ("dup error in"=w33:errorcluster)  [unwired: 8 in, 1 out]
      }
      n108 = while {
        tunnel: w21 -> [w247]
        shift-right: [w251] -> _
        shift-left: T2 {"Status"="", "OsciloscopeClass.lvclass"=refnum} ("Data Cluster") -> [w252]
        tunnel: w25 -> [w255]
        tunnel: [w253] -> w27
        tunnel: w20 -> [w245]
        tunnel: [w244] -> w19
        stop <- w250 stop-if-true
        # "Message Handling Loop"
        n109 = call-dynamic "Delacor_lib_QMH_Dequeue Message.vi"("error in"=w255, "Message Queue in"=w247) -> ("error out"=w254:errorcluster, "Message Data"=w248:variant, "Message"=w249:string, "Message Queue out"=w246:refnum<class "Delacor_lib_QMH_Message Queue.lvclass">)  [unwired: 6 in]
        n110 = case "DQMH_MESSAGE_CASES" shown="\"Read Waveform Osciloscope\"" w249 {
          selector: w249 -> [_ _ _ _ _ _ _ _ _ _ _ _ _ _ _ _ _ w460]
          tunnel: w246 -> [_ _ _ _ _ _ _ _ _ _ _ _ _ _ w411 _ w450 _]
          tunnel: w254 -> [w276 w280 w290 w300 w310 w319 w328 w338 w347 w364 w383 w402 w407 w409 w420 w433 w456 w462]
          tunnel: [w274 w280 w289 w298 w309 w318 w327 w337 w346 w355 w374 w393 w406 w409 w416 w432 w453 w463] -> w256
          tunnel: w252 -> [w267 w279 w284 w299 w304 w314 w321 w332 w341 w351 w370 w389 w405 w408 w415 w430 w449 w461]
          tunnel: [w266 w279 w285 w294 w303 w313 w322 w331 w339 w350 w369 w388 w405 w408 w415 w430 w449 w461] -> w251
          tunnel: [_ _ _ _ _ _ _ _ _ _ _ _ _ _ _ _ w448 _] -> w250
          tunnel: w248 -> [_ _ w288 w297 w308 w317 w326 w336 w345 w362 w381 w400 _ _ w414 _ w446 _]
          tunnel: w245 -> [w262 _ _ _ _ _ _ _ _ _ _ _ _ _ w413 w428 w442 w458]
          tunnel: [_ _ _ _ _ _ _ _ _ _ _ _ _ _ _ _ w444 _] -> w244
          frame "Initialize" {
            w259 = "Initial Message" ("Initial Message")
            # "Initialize - Any operation that needs to be done before the module can receive messages. Synchronize Caller Events.vi will inform Start Module.vi that the module has launched and is ready to receive messages. Module Did Init.vi will broadcast that the module initialized."
            n111 = call "Synchronize Caller Events.vi"("error in (no error)"=w276, "Module Admin"=w262) -> ("error out"=w275:errorcluster, "Module Admin out"=w261:refnum<class "Delacor_lib_QMH_Cloneable Module Admin.lvclass">)  [unwired: 8 in]
            n112 = property class="Mod Admin"(reference=w261) -> ("Accessors:Module ID"=w258:i32, "Accessors:External Launch"=w263:bool)  [unwired: 1 in, 2 out]
            n113 = call "Get Class Instance.vi"() -> ("Classes"=w257:string[])  [unwired: 11 in]
            n114 = call "Module Name--constant.vi"("Module ID"=w258) -> ("Module Name"=w271:string)  [unwired: 10 in]
            n115 = call "Obtain Osciloscope Name.vi"("Osciloscope Class"=w257, "Module ID"=w258) -> ()  [unwired: 9 in, 1 out]
            n116 = property class="VI"("Front Panel.Title"=w271) -> (reference out=w273:refnum<vi>, error out=w278:errorcluster)  [unwired: 2 in]
            n117 = Select(t=T21."Hidden" ("State"), s=w263, f=T21."Standard" ("State")) -> (s? t:f=w268:T21)
            n118 = invoke class="VI" method="FP.Open"(reference=w273, error in=w278, "State"=w268) -> (reference out=w272:refnum<vi>, error out=w277:errorcluster)  [unwired: 2 in, 3 out]
            n119 = call "Module Name--constant.vi"("Module ID"=w258) -> ("Module Name"=w264:string)  [unwired: 10 in]
            n120 = Bundle By Name(cluster=w267, "Status"=w259) -> (w266:T2)
            n121 = invoke class="VI" method="FP.Center"(reference=w272, error in=w277) -> ()  [unwired: 1 in, 3 out]
            n122 = property on="Pane" class="Pane"("Origin"=T20 {"Horizontal"=0, "Vertical"=0}) -> ()  [unwired: 2 in, 2 out]
            n123 = call "Module Did Init.vi"("error in (no error)"=w275, "Initialized?"=TRUE, "Origin"=w264, "Module ID"=w258) -> ("error out"=w274:errorcluster)  [unwired: 7 in]
            "Status" <- w259
          }
          frame "---Module Specific---" {
            # "Separator -- The following cases handle messages specific to this Module."
          }
          frame "Set Com Port" {
            n124 = Variant To Data(error in=w290, type=T5 {"Module ID"=-1, "Com Port"=""} ("Set Com Port Argument"), Variant=w288) -> (data=w286:T5, error out=w289:errorcluster)
            n125 = Unbundle By Name(w284) -> ("OsciloscopeClass.lvclass"=w283:refnum<class "OsciloscopeClass.lvclass">)
            n126 = Unbundle By Name(w286) -> ("Com Port"=w282:refnum<visa-resource-name>)
            n127 = property class="OsciloscopeClass.lvclass"(reference=w283, "Accessors:Com Port"=w282) -> (reference out=w281:refnum<class "OsciloscopeClass.lvclass">)  [unwired: 1 in, 1 out]
            n128 = Bundle By Name(cluster=w284, "OsciloscopeClass.lvclass"=w281) -> (w285:T2)
          }
          frame "Inizializate" {
            n129 = Variant To Data(error in=w300, type=T6 {"Module ID"=-1, "Osciloscope"=""} ("Inizializate Argument"), Variant=w297) -> (data=w295:T6, error out=w298:errorcluster)
            n130 = Unbundle By Name(w295) -> ("Osciloscope"=w293:string)
            n131 = call "Set Class Instance.vi"("Osciloscope Type"=w293) -> ("Obtain Class"=w292:refnum<class "OsciloscopeClass.lvclass">)  [unwired: 10 in]
            n132 = call-dynamic "InitializePort.vi"("OsciloscopeClass in"=w292) -> ("OsciloscopeClass out"=w291:refnum<class "OsciloscopeClass.lvclass">)  [unwired: 9 in, 1 out]
            n133 = Bundle By Name(cluster=w299, "OsciloscopeClass.lvclass"=w291) -> (w294:T2)
          }
          frame "Init Osciloscope" {
            n134 = Variant To Data(error in=w310, type=T7 {"Module ID"=-1, "Boolean"=FALSE, "Initialize--cluster"={"TEKTRONIX-INITIALIZE"={"ID Query? (T: Yes)"=TRUE, "Reset? (T: Yes)"=TRUE, "Serial-Configuration"={"Baud Rate"=9600, "Parity"=0, "Stop Bits"=10, "Flow Control"=2}}, "EDU-X-1200A- INITIALIZE"={"Reset (True)"=TRUE, "ID Query (True)"=TRUE}}} ("Init Osciloscope Argument"), Variant=w308) -> (data=w306:T7, error out=w309:errorcluster)
            n135 = Unbundle By Name(w304) -> ("OsciloscopeClass.lvclass"=w302:refnum<class "OsciloscopeClass.lvclass">)
            n136 = Unbundle By Name(w306) -> ("Initialize--cluster"=w305:T8)
            n137 = call-dynamic "Initialize Osciloscope.vi"("Initialize--cluster"=w305, "OsciloscopeClass in"=w302) -> ("OsciloscopeClass out"=w301:refnum<class "OsciloscopeClass.lvclass">)  [unwired: 8 in, 1 out]
            n138 = Bundle By Name(cluster=w304, "OsciloscopeClass.lvclass"=w301) -> (w303:T2)
          }
          frame "Close Osciloscope" {
            n139 = Unbundle By Name(w314) -> ("OsciloscopeClass.lvclass"=w311:refnum<class "OsciloscopeClass.lvclass">)
            n140 = Variant To Data(error in=w319, type=T9 {"Module ID"=-1, "Boolean"=FALSE} ("Close Osciloscope Argument"), Variant=w317) -> (data=w315:T9, error out=w318:errorcluster)
            n141 = Unbundle By Name(w315) -> ()  [unwired: 2 out]
            n142 = call-dynamic "Close Osciloscope.vi"("OsciloscopeClass in"=w311) -> ("OsciloscopeClass out"=w312:refnum<class "OsciloscopeClass.lvclass">)  [unwired: 9 in, 1 out]
            n143 = Bundle By Name(cluster=w314, "OsciloscopeClass.lvclass"=w312) -> (w313:T2)
          }
          frame "Auto Setup Osciloscope" {
            n144 = Unbundle By Name(w321) -> ("OsciloscopeClass.lvclass"=w323:refnum<class "OsciloscopeClass.lvclass">)
            n145 = Variant To Data(error in=w328, type=T10 {"Module ID"=-1, "Boolean"=FALSE} ("Auto Setup Osciloscope Argument"), Variant=w326) -> (data=w324:T10, error out=w327:errorcluster)
            n146 = Unbundle By Name(w324) -> ()  [unwired: 2 out]
            n147 = call-dynamic "Auto Setup Osciloscope.vi"("OsciloscopeClass in"=w323) -> ("OsciloscopeClass out"=w320:refnum<class "OsciloscopeClass.lvclass">)  [unwired: 9 in, 1 out]
            n148 = Bundle By Name(cluster=w321, "OsciloscopeClass.lvclass"=w320) -> (w322:T2)
          }
          frame "Configure Channel" {
            n149 = Unbundle By Name(w332) -> ("OsciloscopeClass.lvclass"=w329:refnum<class "OsciloscopeClass.lvclass">)
            n150 = Variant To Data(error in=w338, type=T11 {"Module ID"=-1, "Configurate Channel--cluster"={"Tektronix"={"Enable Channel (True)"=TRUE, "Channel (0: Channel 1)"=0, "Vertical Coupling (1: DC)"=1, "Probe Attenuation (10: 10X)"=10, "Vertical Range (10.0 V/div)"=10.0, "Vertical Offset (0.0 divs)"=0.0, "Bandwidth (0: MAX Bandwidth)"=0}, "EDU-X-1002A"={"Vertical Scale (5.0 V)"=5.0, "Impedance (0: 1 MOhm)"=0, "Channel Name (0: Channel 1)"=0, "Coupling (1: DC)"=1, "Vertical Range (40.0 V)"=40.0, "Vertical Offset (0.0)"=0.0, "Probe Attenuation (1.0)"=1.0, "Vertical Setting (1: Vertical Range)"=1}}} ("Configure Channel Argument"), Variant=w336) -> (data=w334:T11, error out=w337:errorcluster)
            n151 = Unbundle By Name(w334) -> ("Configurate Channel--cluster"=w333:T12)
            n152 = call-dynamic "Configurate Channel Osciloscope.vi"("Configurate Channel--cluster"=w333, "OsciloscopeClass in"=w329) -> ("OsciloscopeClass out"=w330:refnum<class "OsciloscopeClass.lvclass">)  [unwired: 8 in, 1 out]
            n153 = Bundle By Name(cluster=w332, "OsciloscopeClass.lvclass"=w330) -> (w331:T2)
          }
          frame "Reset Osciloscope" {
            n154 = Unbundle By Name(w341) -> ("OsciloscopeClass.lvclass"=w342:refnum<class "OsciloscopeClass.lvclass">)
            n155 = Variant To Data(error in=w347, type=T13 {"Module ID"=-1, "Boolean"=FALSE} ("Reset Osciloscope Argument"), Variant=w345) -> (data=w343:T13, error out=w346:errorcluster)
            n156 = Unbundle By Name(w343) -> ()  [unwired: 2 out]
            n157 = call-dynamic "Reset Osciloscope.vi"("OsciloscopeClass in"=w342) -> ("OsciloscopeClass out"=w340:refnum<class "OsciloscopeClass.lvclass">)  [unwired: 9 in, 1 out]
            n158 = Bundle By Name(cluster=w341, "OsciloscopeClass.lvclass"=w340) -> (w339:T2)
          }
          frame "Read Waveform Osciloscope" {
            n159 = Unbundle By Name(w351) -> ("OsciloscopeClass.lvclass"=w352:refnum<class "OsciloscopeClass.lvclass">)
            n160 = Variant To Data(error in=w364, type=T14 {"Module ID"=-1, "ReadWaveform"={"TEKTRONIX READ-WAVEFORM 2"={"Source (0: Channel 1)"=0, "Timeout (10000 ms) 2"=10000}, "EDU-X-1200A- READ-WAVEFORM"={"Bind Source Channel (2: None)"=2, "Timeout (10000 ms)"=10000, "Source Channel (0: Channel 1)"=0}}, "Wait Notifier"=refnum, "wait for reply"=FALSE} ("Read Waveform Osciloscope Argument"), Variant=w362) -> (data=w360:T14, error out=w363:errorcluster)
            n161 = Unbundle By Name(w360) -> ("ReadWaveform"=w353:T15, "Wait Notifier"=w359:refnum<notifier>, "wait for reply"=w358:bool)
            n162 = call-dynamic "Read Waveform Osciloscope.vi"("ReadWaveform"=w353, "OsciloscopeClass in"=w352) -> ("error out"=w348:errorcluster, "Waveform Data"=w354:waveform(dbl), "OsciloscopeClass out"=w349:refnum<class "OsciloscopeClass.lvclass">)  [unwired: 7 in]
            n163 = Bundle By Name(cluster=T22 {"Waveform Graph"=[], "Read Waveform Osciloscope_error"={"status"=FALSE, "code"=0, "source"=""}} ("Read Waveform Osciloscope (Reply Payload)"), "Waveform Graph"=w354) -> (w357:T22)
            n164 = Merge Errors(w363, w348) -> (w355:errorcluster)
            n165 = Bundle By Name(cluster=w351, "OsciloscopeClass.lvclass"=w349) -> (w350:T2)
            n166 = case shown="True" w358 {
              tunnel: w359 -> [_ w366]
              tunnel: w357 -> [_ w365]
              frame False {
              }
              frame True {
                n167 = Send Notification(notification=w365, notifier=w366) -> ()  [unwired: 1 in, 2 out]
              }
            }
          }
          frame "Read Measurement Osciloscope" {
            n168 = Unbundle By Name(w370) -> ("OsciloscopeClass.lvclass"=w371:refnum<class "OsciloscopeClass.lvclass">)
            n169 = Variant To Data(error in=w383, type=T16 {"Module ID"=-1, "Read Measurement In"={"TEKTRONIX- READ-IN"={"Channel (1: Channel 1)"=1, "Measurement Type (0: Frequency)"=0}, "EDU-X-1200A- READ-IN"={"Slope Type (0: Positive)"=0, "Measurement Type (0: Peak-Peak)"=0, "Occurrence Value (1)"=1, "Vertical Cross Value (0)"=0.0}}, "Wait Notifier"=refnum, "wait for reply"=FALSE} ("Read Measurement Osciloscope Argument"), Variant=w381) -> (data=w379:T16, error out=w382:errorcluster)
            n170 = Unbundle By Name(w379) -> ("Read Measurement In"=w372:T17, "Wait Notifier"=w378:refnum<notifier>, "wait for reply"=w377:bool)
            n171 = call-dynamic "Read Measurement Osciloscope.vi"("Read Measurement In"=w372, "OsciloscopeClass in"=w371) -> ("error out"=w367:errorcluster, "Read measurement Out"=w373:T24, "OsciloscopeClass out"=w368:refnum<class "OsciloscopeClass.lvclass">)  [unwired: 7 in]
            n172 = Merge Errors(w382, w367) -> (w374:errorcluster)
            n173 = Bundle By Name(cluster=T23 {"Read measurement Out"={"Tektronix-1200A-READ-OUT"={"Units"="", "Measurement"=0.0}, "EDU-X-1200A- READ-OUT"={"Measurement"=0.0}}, "Read Measurement Osciloscope_error"={"status"=FALSE, "code"=0, "source"=""}} ("Read Measurement Osciloscope (Reply Payload)"), "Read measurement Out"=w373) -> (w376:T23)
            n174 = Bundle By Name(cluster=w370, "OsciloscopeClass.lvclass"=w368) -> (w369:T2)
            n175 = case shown="True" w377 {
              tunnel: w378 -> [_ w385]
              tunnel: w376 -> [_ w384]
              frame False {
              }
              frame True {
                n176 = Send Notification(notification=w384, notifier=w385) -> ()  [unwired: 1 in, 2 out]
              }
            }
          }
          frame "Read 2 Measurement Channels Osciloscope" {
            n177 = Variant To Data(error in=w402, type=T18 {"Module ID"=-1, "Read 2 channels In"={"TEKTRONIX- READ-CHANNELS-IN"={"Channel 1 (1: Channel 1)"=1, "Channel 2 (2: Channel 2)"=2, "Measurement Type (0: Phase)"=0}, "EDU-X-1200A- READ-CHANNELS-IN"={"Timeout (10000 ms)"=10000, "Channels"=[]}}, "Wait Notifier"=refnum, "wait for reply"=FALSE} ("Read 2 Measurement Channels Osciloscope Argument"), Variant=w400) -> (data=w398:T18, error out=w401:errorcluster)
            n178 = Unbundle By Name(w389) -> ("OsciloscopeClass.lvclass"=w390:refnum<class "OsciloscopeClass.lvclass">)
            n179 = Unbundle By Name(w398) -> ("Read 2 channels In"=w391:T19, "Wait Notifier"=w397:refnum<notifier>, "wait for reply"=w396:bool)
            n180 = call-dynamic "Read 2 measurement Channels Osciloscope.vi"("Read 2 channels In"=w391, "OsciloscopeClass in"=w390) -> ("error out"=w386:errorcluster, "Read 2 channels Out"=w392:T26, "OsciloscopeClass out"=w387:refnum<class "OsciloscopeClass.lvclass">)  [unwired: 7 in]
            n181 = Merge Errors(w401, w386) -> (w393:errorcluster)
            n182 = Bundle By Name(cluster=T25 {"Read 2 channels Out"={"TEKTRONIX READ-CHANNELS-OUT "={"Units"="", "Measurement"=0.0}, "EDU-X-1200A- READ-CHANNELS-OUT"={"Measurements"=[]}}, "Read 2 Measurement Channels Osciloscope_error"={"status"=FALSE, "code"=0, "source"=""}} ("Read 2 Measurement Channels Osciloscope (Reply Payload)"), "Read 2 channels Out"=w392) -> (w395:T25)
            n183 = Bundle By Name(cluster=w389, "OsciloscopeClass.lvclass"=w387) -> (w388:T2)
            n184 = case shown="True" w396 {
              tunnel: w397 -> [_ w404]
              tunnel: w395 -> [_ w403]
              frame False {
              }
              frame True {
                n185 = Send Notification(notification=w403, notifier=w404) -> ()  [unwired: 1 in, 2 out]
              }
            }
          }
          frame "---Copy This Frame---" {
            # "Duplicate this frame when creating new messages.  Change this comment in the duplicated frame to describe this message."
            n186 = Merge Errors(w407) -> (w406:errorcluster)
          }
          frame "---Exit and Error Handling---" {
            # "Separator - the following cases handle errors and exit messages."
          }
          frame "Error" {
            # "#CodeRecommended - If you ever change the name of this \"Error\" message, you'll need to update the name in the Check Loop Error.vi as well."
            # "#CodeRecommended - If the module is running in standalone mode (External Launch = FALSE), this code will pop up an error dialog and call the 'Exit' message if an error occurs. Add more fine-grained error handling here."
            # "Error - Check the error message data and respond accordingly. This message is sent by the \"Error Handler\" VIs at the end of each loop in this application."
            n187 = property class="Mod Admin"(reference=w413) -> ("Accessors:External Launch"=w412:bool, "Accessors:Module ID"=w410:i32)  [unwired: 1 in, 2 out]
            n188 = Variant To Data(error in=w420, type=errorcluster {"status"=FALSE, "code"=0, "source"=""} ("error constant"), Variant=w414) -> (data=w421:errorcluster, error out=w418:errorcluster)
            n189 = call "Error Reported.vi"("Error"=w421, "Module ID"=w410) -> ()  [unwired: 9 in, 1 out]
            n190 = case shown="False" w412 {
              tunnel: [w426 _] -> w417
              tunnel: w411 -> [w424 _]
              tunnel: w421 -> [w425 _]
              frame False {
                # "If the module is running standalone, then pop up an error dialog and call the \"Exit\" message."
                n191 = call <vilib>:"Simple Error Handler.vi"("error in (no error)"=w425) -> ()  [unwired: 4 in, 5 out]
                n192 = call-poly <vilib>:"Delacor_lib_QMH_Enqueue Message (poly).vi"("Priority Message? (F)"=TRUE, "Message"="Exit", "Message Queue in"=w424) -> ("error out"=w426:errorcluster)  [unwired: 7 in, 1 out]
              }
              frame True {
                # "If the module was launched externally, calling the Error Reported broadcast VI is the only action performed by the \"Error\" message. The module's caller can then process the error appropriately."
              }
            }
            n193 = Merge Errors(w418, w417) -> (w416:errorcluster)
            n194 = local write "error out"(w416) -> ()
          }
          frame "Simulate MHL Error" {
            # "#DQMH_HowTo The 'Simulate MHL Error' button  illustrates how the MHL handles errors. This event is instructional in nature and can be removed."
            # "Simulate an error occurring at the MHL"
            n195 = property class="Mod Admin"(reference=w428) -> ("Accessors:Module ID"=w429:i32)  [unwired: 1 in, 2 out]
            n196 = call "Module Name--constant.vi"("Module ID"=w429) -> ("Module Name"=w427:string)  [unwired: 10 in]
            n197 = xnode "Error Ring"("parameter 0"=w427) -> ("error out"=w431:errorcluster)
            n198 = Merge Errors(w433, w431) -> (w432:errorcluster)
          }
          frame "Exit" {
            w447 = 91  # 91: not all Exit messages will have an argument
            w448 = TRUE  # Stop the VI
            # "Release the message queue reference"
            # "#CodeNeeded - Add any required cleanup code here."
            # "Exit - Exit the application."
            n199 = Variant To Data(error in=w456, type=T4 {"Module ID"=-1, "Origin"="", "Exit via Stop Module Req?"=FALSE, "Wait for Module to stop?"=FALSE} ("Stop Argument"), Variant=w446) -> (data=w443:T4, error out=w451:errorcluster)
            n200 = call <vilib>:"Clear Errors.vi"("error in (no error)"=w451, "specific error code to clear (0: all)"=w447) -> ("error out"=w455:errorcluster)  [unwired: 4 in, 1 out]
            n201 = control-ref of="This VI"() -> (w441:refnum<vi>)
            n202 = call-dynamic "Delacor_lib_QMH_Release Message Queue.vi"("error in"=w455, "Message Queue"=w450) -> ("error out"=w454:errorcluster)  [unwired: 9 in]
            n203 = call "Handle Exit.vi"("Stop Argument"=w443, "Module Admin in"=w442, "VI reference"=w441) -> ("error out"=w452:errorcluster, "Wait for Stop?"=w444:bool)  [unwired: 7 in]
            n204 = Merge Errors(w454, w452) -> (w453:errorcluster)
          }
          frame Default {
            # "'Default' case only runs if there is a message that isn't defined in any of the other cases.  Output a programming error."
            n205 = property class="Mod Admin"(reference=w458) -> ("Accessors:Module ID"=w457:i32)  [unwired: 1 in, 2 out]
            n206 = call "Module Name--constant.vi"("Module ID"=w457) -> ("Module Name"=w459:string)  [unwired: 10 in]
            n207 = xnode "Error Ring"("parameter 0"=w460, "parameter 1"=w459) -> ("error out"=w464:errorcluster)
            n208 = Merge Errors(w462, w464) -> (w463:errorcluster)
          }
        }
        n209 = call-dynamic "Delacor_lib_QMH_Error Handler - Message Handling Loop.vi"("error in"=w256, "Message Queue in"=w246) -> ("dup error in"=w253:errorcluster)  [unwired: 8 in, 1 out]
      }
    }
    frame Error {
      n210 = call "Synchronize Caller Events.vi"("Module Admin"=w478) -> ("Module Admin out"=w477:refnum<class "Delacor_lib_QMH_Cloneable Module Admin.lvclass">)  [unwired: 9 in, 1 out]
      n211 = property class="Mod Admin"(reference=w477) -> ("Accessors:Module ID"=w476:i32)  [unwired: 1 in, 2 out]
      n212 = call-dynamic "Delacor_lib_QMH_Release Message Queue.vi"("error in"=w475, "Message Queue"=w473) -> ("error out"=w474:errorcluster)  [unwired: 9 in]
      n213 = call "Module Name--constant.vi"("Module ID"=w476) -> ("Module Name"=w481:string)  [unwired: 10 in]
      n214 = Format Into String(format string="An error occurred during initialization. %s is no longer running.", w481) -> (resulting string=w479:string)  [unwired: 2 in, 1 out]
      n215 = call "Error Reported.vi"("Additional Information"=w479, "Error"=w474, "Module ID"=w476) -> ()  [unwired: 8 in, 1 out]
    }
  }
  n216 = Merge Errors(w17, w16) -> (w18:errorcluster)
  n217 = call "Close Module.vi"("error in"=w18, "Wait for stop?"=w2, "Module Admin in"=w4) -> ("error out"=w14:errorcluster, "External Launch"=w1:bool, "Module Admin out"=w3:refnum<class "Delacor_lib_QMH_Cloneable Module Admin.lvclass">)  [unwired: 6 in]
  n218 = Unregister For Events(event registration refnum=w9, error in=w14) -> (error out=w13:errorcluster)
  "error out" <- w13
  n219 = local write "Module Admin"(w3) -> ()
  n220 = case "External Launch?" shown="True" w1 {
    tunnel: w13 -> [_ w483]
    frame False {
    }
    frame True {
      n221 = case shown="No Error" w483 {
        frame No Error {
          n222 = invoke class="VI" method="FP.Close"() -> ()  [unwired: 3 in, 3 out]
        }
        frame Error {
          n223 = invoke class="VI" method="FP.Open"("Activate"=TRUE ("Activate?")) -> ()  [unwired: 4 in, 5 out]
        }
      }
    }
  }
